vi "Do.vi"(8 "error in (no error)":errorcluster, 10 "Actor in":refnum<class "Actor.lvclass">, 11 "Configure RangeMax Msg":refnum<class "Configure RangeMax Msg.lvclass">) -> (0 "error out":errorcluster, 2 "Actor out":refnum<class "Actor.lvclass">)   [LabVIEW 2015, in "CS++Motor.lvlib" / "Configure RangeMax Msg.lvclass"]
doc: "This VI delivers the message to the actor by calling the appropriate method(s) on the actor."
uses:
  Configure RangeMax Msg.lvclass
  CS++Motor/CS++Motor.lvclass
  CSPP_Core/Actors/CS++PVMonitor Messages/CS++PVUpdate Msg/CS++PVUpdate Msg.lvclass
  CSPP_Core/Classes/CS++ProcessVariables/ProcessVariable/PV.lvclass
  <vilib>/ActorFramework/Actor/Actor.lvclass
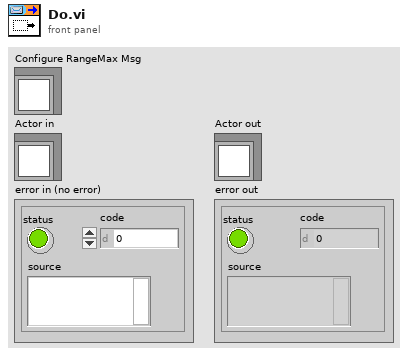
[diagram p1: front panel]
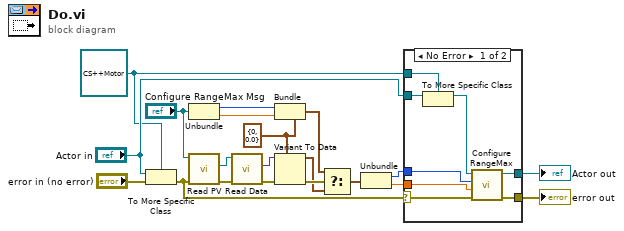
[diagram p0: block diagram]
diagram:
  w12 = cluster{"AxisNumber":u8, "RangeMax":dbl} {"AxisNumber"=0, "RangeMax"=0.0} ("Type")
  w16 = refnum<class "CS++Motor.lvclass"> refnum ("Actor in")
  n1 = To More Specific Class(target class=w16, reference="Actor in", error in="error in (no error)") -> (error out=w5:errorcluster)  [unwired: 1 out]
  n2 = Unbundle ("Pre-Unbundler")("Configure RangeMax Msg") -> (w2:u8, w1:dbl)
  n3 = call "Read PV.vi"("error in (no error)"=w5, "CS++PVUpdate Msg in"="Configure RangeMax Msg") -> ("error out"=w15:errorcluster, "PV"=w11:refnum<class "PV.lvclass">)  [unwired: 7 in, 1 out]
  n4 = call "Read Data.vi"("error in (no error)"=w15, "PV in"=w11) -> ("error out"=w9:errorcluster, "Data"=w10:variant)  [unwired: 7 in, 1 out]
  n5 = Bundle ("Pre-Bundler")(cluster=w12, "AxisNumber"=w2, "RangeMax"=w1) -> (w13:cluster{"AxisNumber":u8, "RangeMax":dbl})
  n6 = Variant To Data(error in=w9, type=w12, Variant=w10) -> (data=w7:cluster{"AxisNumber":u8, "RangeMax":dbl}, error out=w14:errorcluster)
  n7 = Select ("MainSelect")(t=w13, s=w14, f=w7) -> (s? t:f=w8:cluster{"AxisNumber":u8, "RangeMax":dbl})
  n8 = Unbundle ("Main-Unbundler")(w8) -> ("AxisNumber"=w4:u8, "RangeMax"=w3:dbl)
  n9 = case shown="No Error" w5 {
    selector: w5 -> [w26 w30]
    tunnel: [w28 w30] -> w19
    tunnel: [w27 w29] -> w18
    tunnel: "Actor in" -> [w25 w29]
    tunnel: w16 -> [w24 _]
    tunnel: w4 -> [w22 _]
    tunnel: w3 -> [w21 _]
    frame No Error {
      n10 = To More Specific Class(target class=w24, reference=w25) -> (specific class reference=w23:refnum<class "CS++Motor.lvclass">)  [unwired: 1 in, 1 out]
      n11 = call "Configure RangeMax.vi"("error in (no error)"=w26, "RangeMax"=w21, "AxisNumber"=w22, "CS++Motor in"=w23) -> ("error out"=w28:errorcluster, "CS++Motor out"=w27:refnum<class "CS++Motor.lvclass">)  [unwired: 6 in]
    }
    frame Error {
    }
  }
  "error out" <- w19
  "Actor out" <- w18
